vi "SJ_ODE_RHS_DISP.vi"(2 "data":T1, 3 "t":dbl, 4 "x":dbl[](array[numeric])) -> (0 "error out":errorcluster, 1 "f(x,t)":dbl[](array[numeric]))   [LabVIEW 2012]
doc: "This template is the starting point for creating a function that is the right-hand-side of an ordinary differential equaltion to be passed to the ODE Solver.vi."
uses:
  <vilib>/gmath/NumericalOptimization/objective function data.ctl
  SJ_ODE_Data.ctl
  Utilities/fluid_properties/fluid_types.ctl
  LEM_Solution_Controls.ctl
  Model.ctl
  Fourier_Series.ctl
  Utilities/fluid_properties/fluid_properties.ctl
  <vilib>/gmath/NI_Gmath.lvlib
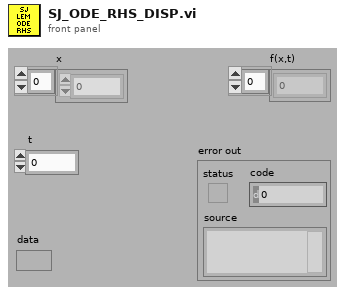
[diagram p1: front panel]
types:
  T1 = typedef "NI_Gmath.lvlib/objective function data.ctl" = variant
  T2 = typedef "SJ_ODE_Data.ctl" = cluster{"Fluid Properties":cluster{"Fluid":T3, "Temperature (K)":dbl, "Pressure (Pa)":dbl}, "SJ Geometry":cluster{"Do (mm)":dbl, "Ho (mm)":dbl, "Dc (mm)":dbl, "Hc (mm)":dbl}, "Solution Controls":T4, "Misc Data":cluster{"Freq jet":dbl, "Coefficients":dbl[], "Nat Frequ":dbl, "Ku":dbl, "Scale":dbl, "Fourier Series":T6, "Km":dbl, "Kr":dbl}, "Thermo and Transport Properties":T7, "LEM Output Data":cluster{"X":dbl[][], "times":dbl[], "|X|":dbl, "PA X":dbl}}
  T3 = typedef "fluid_types.ctl" = enum16{"Air", "Water"}
  T4 = typedef "LEM_Solution_Controls.ctl" = cluster{"Simulation":enum16{"Sinusoidal", "Fourier Series"}, "Fixed Parameter":enum16{"Pressure", "Displacement"}, "Model":T5, "# time steps":i32, "# periods":i32, "Tolerance":dbl, "STFT periods":i32}
  T5 = typedef "Model.ctl" = enum16{"Martin", "Tang", "Gallas", "Persoon"}
  T6 = typedef "Fourier_Series.ctl" = cluster{"Amp":dbl, "Phase":dbl}[]
  T7 = typedef "fluid_properties.ctl" = cluster{"nu":dbl, "c":dbl, "Pr":dbl, "Cp":dbl, "Cv":dbl, "gamma":dbl, "mu":dbl, "rho":dbl}
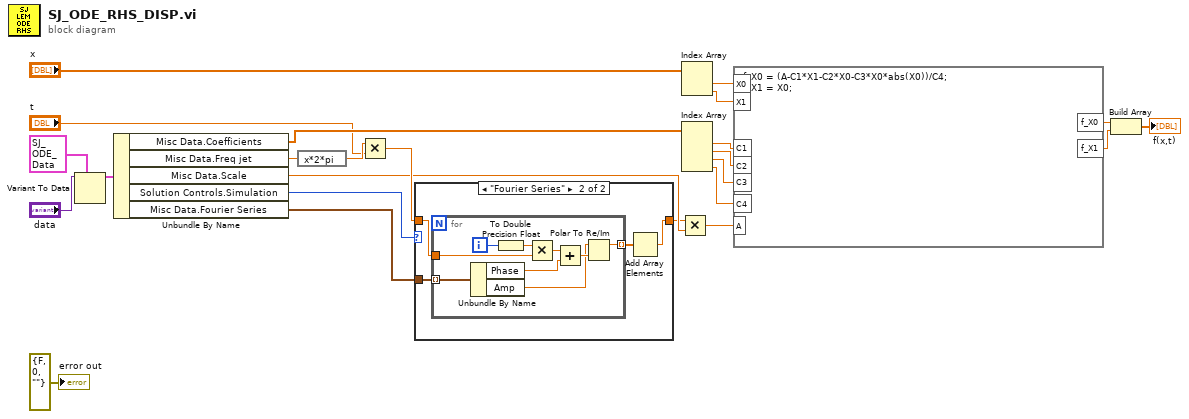
[diagram p0: block diagram]
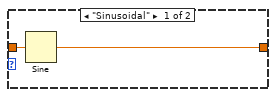
[diagram p2: hidden frame]
diagram:
  n1 = Variant To Data(type=T2 {"Fluid Properties"={"Fluid"=enum."Air", "Temperature (K)"=0.0, "Pressure (Pa)"=0.0}, "SJ Geometry"={"Do (mm)"=0.0, "Ho (mm)"=0.0, "Dc (mm)"=0.0, "Hc (mm)"=0.0}, "Solution Controls"={"Simulation"=enum."Sinusoidal", "Fixed Parameter"=enum."Pressure", "Model"=enum."Tang", "# time steps"=0, "# periods"=0, "Tolerance"=0.0, "STFT periods"=0}, "Misc Data"={"Freq jet"=0.0, "Coefficients"=[], "Nat Frequ"=0.0, "Ku"=0.0, "Scale"=0.0, "Fourier Series"=[], "Km"=0.0, "Kr"=0.0}, "Thermo and Transport Properties"={"nu"=0.0, "c"=0.0, "Pr"=0.0, "Cp"=0.0, "Cv"=0.0, "gamma"=0.0, "mu"=0.0, "rho"=0.0}, "LEM Output Data"={"X"=[], "times"=[], "|X|"=0.0, "PA X"=0.0}} ("ODE Data"), Variant="data") -> (data=w22:T2)  [unwired: 1 in, 1 out]
  n2 = Unbundle By Name(w22) -> ("Misc Data.Coefficients"=w16:dbl[], "Misc Data.Freq jet"=w9:dbl, "Misc Data.Scale"=w5:dbl, "Solution Controls.Simulation"=w4:enum16{"Sinusoidal", "Fourier Series"}, "Misc Data.Fourier Series"=w2:T6)
  n3 = expression code="x*2*pi"(w9) -> (w8:dbl)
  n4 = Multiply(x=w8, y="t") -> (x*y=w6:dbl)
  n5 = case shown="\"Fourier Series\"" w4 {
    tunnel: w6 -> [w26 w29]
    tunnel: [w25 w27] -> w1
    tunnel: w2 -> [_ w30]
    frame "Sinusoidal" {
      n6 = Sine(x=w26) -> (sin(x)=w25:dbl)
    }
    frame "Fourier Series" {
      n7 = for {
        tunnel: w30 -> [w37] mode=indexing
        tunnel: w29 -> [w38]
        tunnel: [w32] -> w28 mode=indexing
        i -> [w33]
        n8 = Unbundle By Name(w37) -> ("Phase"=w35:dbl, "Amp"=w31:dbl)
        n9 = To Double Precision Float(number=w33) -> (double precision float=w39:dbl)
        n10 = Multiply(x=w39, y=w38) -> (x*y=w36:dbl)
        n11 = Add(x=w36, y=w35) -> (x+y=w34:dbl)
        n12 = Polar To Re/Im(2:w34, 3:w31) -> (1:w32:dbl)  [unwired: 1 out]
      }
      n13 = Add Array Elements(numeric array=w28) -> (sum=w27:dbl)
    }
  }
  n14 = Multiply(x=w1, y=w5) -> (x*y=w3:dbl)
  n15 = Index Array(array="x") -> (element #1=w19:dbl, element #2=w11:dbl)  [unwired: 2 in]
  n16 = Index Array(array=w16) -> (element #1=w15:dbl, element #2=w14:dbl, element #3=w13:dbl, element #4=w12:dbl)  [unwired: 4 in]
  n17 = formula code="f_X0 = (A-C1*X1-C2*X0-C3*X0*abs(X0))/C4;\nf_X1 = X0;"("C1"=w15, "C2"=w14, "C3"=w13, "X0"=w19, "A"=w3, "C4"=w12, "X1"=w11) -> ("f_X0"=w18:dbl, "f_X1"=w10:dbl)
  n18 = Build Array(w18, w10) -> (→"f(x,t)":dbl[])
  "error out" <- errorcluster {"status"=FALSE, "code"=0, "source"=""} ("error out")
